vi "超标留样启动流程.vi"   [LabVIEW 2016, in "德润DR803F超标留样.lvlib"]
types:
  T1 = cluster{"工作状态":u16, "工作进程":u16, "仪器时间":timestamp, "采样模式":u16, "当前瓶号":dbl, "采样瓶数":dbl, "每瓶采样次数":dbl, "当前瓶已采次数":dbl, "当前瓶采样量":dbl, "采样量定量":dbl, "采样量比例":dbl, "瞬时流量":dbl, "累积流量":dbl, "外置泵状态":dbl, "采样泵状态":dbl, "采样泵方向":dbl, "采样阀":dbl, "采样瓶转盘":dbl, "排水阀":dbl, "清洗泵":dbl, "清洗管工作":dbl, "清洗管电源":dbl, "清洗管运行方向":dbl, "门状态":u16, "采水管有水检测":dbl}
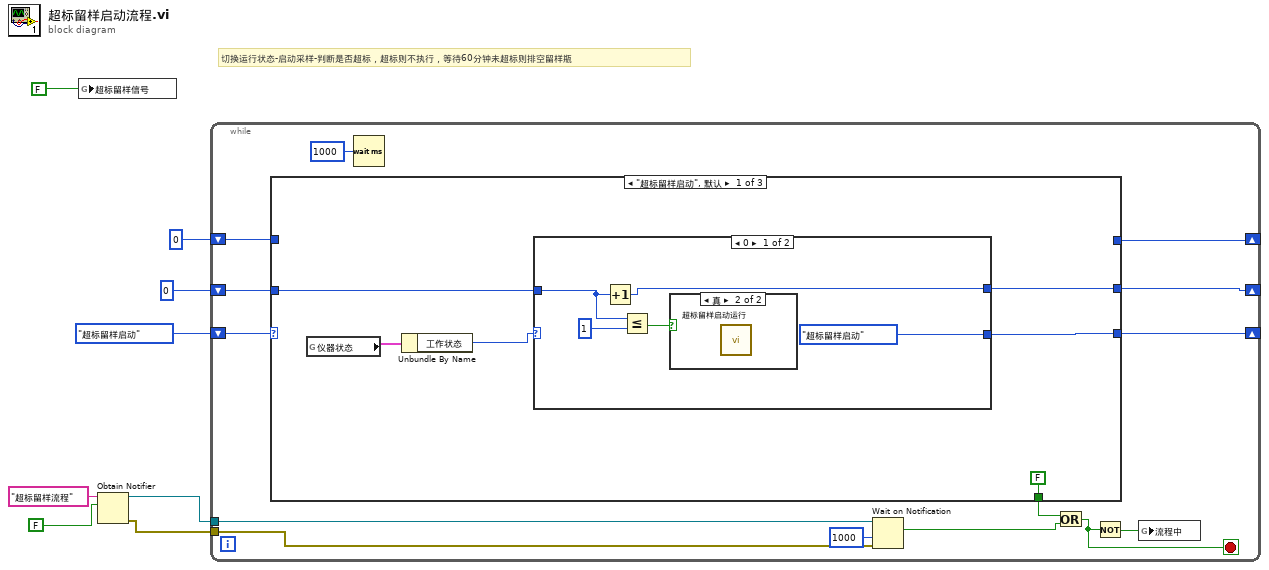
[diagram p0: block diagram]
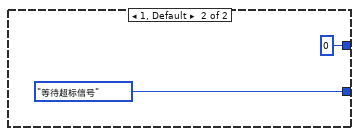
[diagram p3: hidden frame]
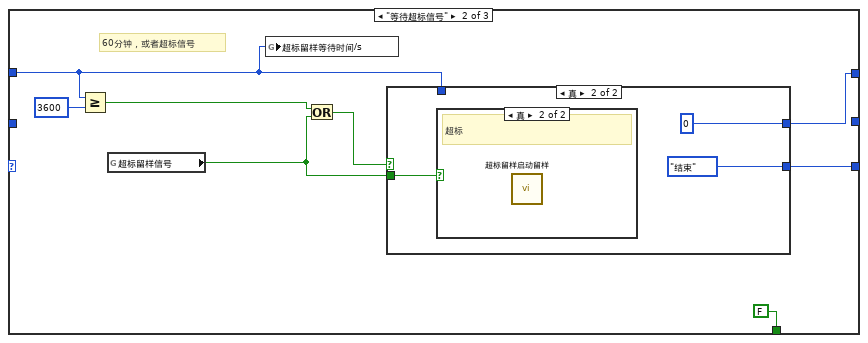
[diagram p4: hidden frame]
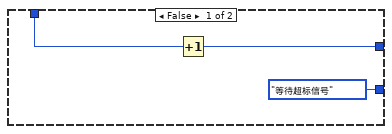
[diagram p5: hidden frame]
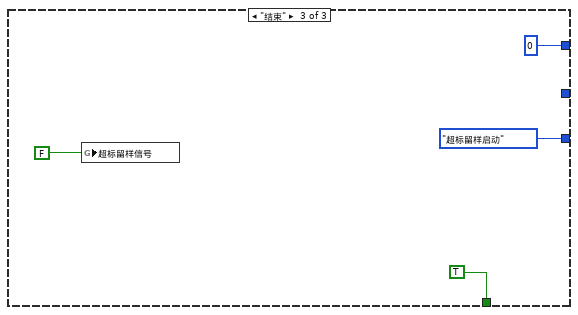
[diagram p7: hidden frame]
diagram:
  # "切换运行状态-启动采样-判断是否超标，超标则不执行，等待60分钟未超标则排空留样瓶"
  n1 = global write "超标留样全局.vi" "超标留样信号"(FALSE ("采样完成")) -> ()
  n2 = Obtain Notifier(name (unnamed)="超标留样流程" ("名称（未命名）"), notification data type=FALSE ("采样完成")) -> (notifier out=w4:refnum<notifier>, error out=w3:errorcluster)  [unwired: 2 in, 1 out]
  n3 = while {
    shift-right: [w12] -> _
    shift-left: enum16{"超标留样启动", "等待超标信号", "结束"}."超标留样启动" -> [w22]
    shift-right: [w19] -> _
    shift-left: 0 -> [w20]
    tunnel: w4 -> [w18]
    tunnel: w3 -> [w17]
    shift-right: [w9] -> _
    shift-left: 0 -> [w10]
    stop <- w15 stop-if-true
    n4 = case shown="\"超标留样启动\", 默认" w22 {
      tunnel: w20 -> [_ w36 _]
      tunnel: [_ w41 0] -> w19
      tunnel: [w25 w39 enum16{"超标留样启动", "等待超标信号", "结束"}."超标留样启动"] -> w12
      tunnel: [FALSE FALSE TRUE] -> w11
      tunnel: w10 -> [w24 _ _]
      tunnel: [w23 _ _] -> w9
      frame "超标留样启动", Default {
        n5 = global read "超标留样全局.vi" "仪器状态"() -> (w28:T1)
        n6 = Unbundle By Name(w28) -> ("工作状态"=w26:u16)
        n7 = case shown="0" w26 {
          tunnel: [enum16{"超标留样启动", "等待超标信号", "结束"}."超标留样启动" enum16{"超标留样启动", "等待超标信号", "结束"}."等待超标信号"] -> w25
          tunnel: w24 -> [w30 _]
          tunnel: [w29 0] -> w23
          frame 0 {
            n8 = Increment(x=w30) -> (x+1=w29:i32)
            n9 = Less Or Equal?(x=w30, y=1) -> (x <= y?=w31:bool)
            n10 = case shown="真" w31 {
              frame False {
              }
              frame True {
                n11 = call "超标留样启动运行.vi"() -> ()  [unwired: 11 in, 1 out]
              }
            }
          }
          frame 1, Default {
          }
        }
      }
      frame "等待超标信号" {
        # "60分钟，或者超标信号"
        n12 = Greater Or Equal?(x=w36, y=3600) -> (x >= y?=w42:bool)
        n13 = global read "超标留样全局.vi" "超标留样信号"() -> (w38:bool)
        n14 = global write "超标留样全局.vi" "超标留样等待时间/s"(w36) -> ()
        n15 = Or(x=w42, y=w38) -> (x .or. y?=w40:bool)
        n16 = case shown="真" w40 {
          tunnel: [enum16{"超标留样启动", "等待超标信号", "结束"}."等待超标信号" enum16{"超标留样启动", "等待超标信号", "结束"}."结束"] -> w39
          tunnel: w36 -> [w46 _]
          tunnel: [w45 0] -> w41
          tunnel: w38 -> [_ w47]
          frame False {
            n17 = Increment(x=w46) -> (x+1=w45:i32)
          }
          frame True {
            n18 = case shown="真" w47 {
              frame False {
                # "超时但不超标"
              }
              frame True {
                # "超标"
                n19 = call "超标留样启动留样.vi"() -> ()  [unwired: 11 in, 1 out]
              }
            }
          }
        }
      }
      frame "结束" {
        n20 = global write "超标留样全局.vi" "超标留样信号"(FALSE ("采样完成")) -> ()
      }
    }
    n21 = Wait (ms)(milliseconds to wait=u32 1000 ("等待时间（毫秒）")) -> ()  [unwired: 1 out]
    n22 = Wait on Notification(notifier=w18, timeout in ms (-1)=1000 ("超时毫秒(-1)"), error in (no error)=w17) -> (notification=w14:bool)  [unwired: 1 in, 3 out]
    n23 = Or(x=w11, y=w14) -> (x .or. y?=w15:bool)
    n24 = Not(x=w15) -> (.not. x?=w13:bool)
    n25 = global write "超标留样全局.vi" "流程中"(w13) -> ()
  }
